vi "Register for gRPC Server Events.vi"(8 "error in (no error)":errorcluster, 11 "CIFLauncher in":refnum<class "CIFPluginLoader.lvclass">) -> (0 "error out":errorcluster, 1 "Abort VI Event Registration Refnum":refnum<event-registration>, 2 "Main Event Registration Refnum":refnum<event-registration>, 3 "CIFLauncher out":refnum<class "CIFPluginLoader.lvclass">, 4 "Discovery Event Registration Refnum":refnum<event-registration>)   [LabVIEW 2021, in "CIFPluginLoader.lvclass"]
uses:
  CIFPluginLoader.lvclass
  <vilib>/gRPC/LabVIEW gRPC Library/Server API/typeDefs/gRPCId Cluster.ctl
  <vilib>/gRPC/LabVIEW gRPC Library/Shared/grpcId.ctl
  CIFPluginLoader.lvclass/CIFPluginLoader.ctl
  CIF_PluginLoader_server/RPC Service/PluginLoader/PluginLoader.lvclass/PluginLoader.ctl
  CIF_PluginLoader_server/RPC Service/PluginLoader/PluginLoader.lvclass
  <vilib>/gRPC/LabVIEW gRPC Library/grpc-lvsupport-release.lvlib
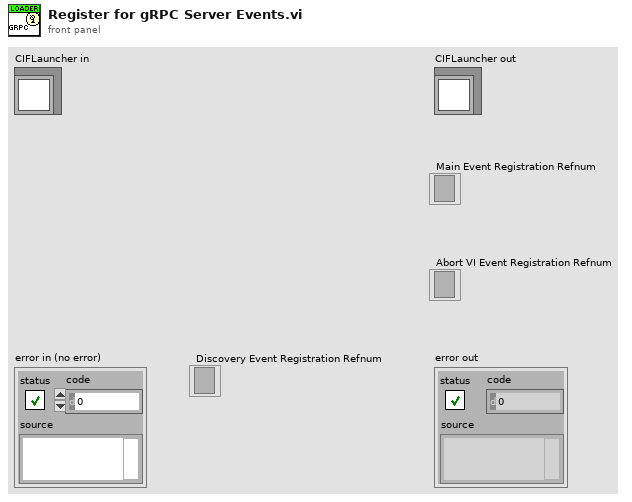
[diagram p1: front panel]
types:
  T1 = typedef "CIF_PluginLoader_server.lvlib/PluginLoader.lvclass/Server gRPC UEs.ctl" = cluster{"PluginLoader LoadPlugin gRPC UE":refnum<user-event>, "PluginLoader AbortPlugin gRPC UE":refnum<user-event>, "PluginLoader Destroy gRPC UE":refnum<user-event>, "PluginLoader Ping gRPC UE":refnum<user-event>, "PluginLoader Discover gRPC UE":refnum<user-event>}
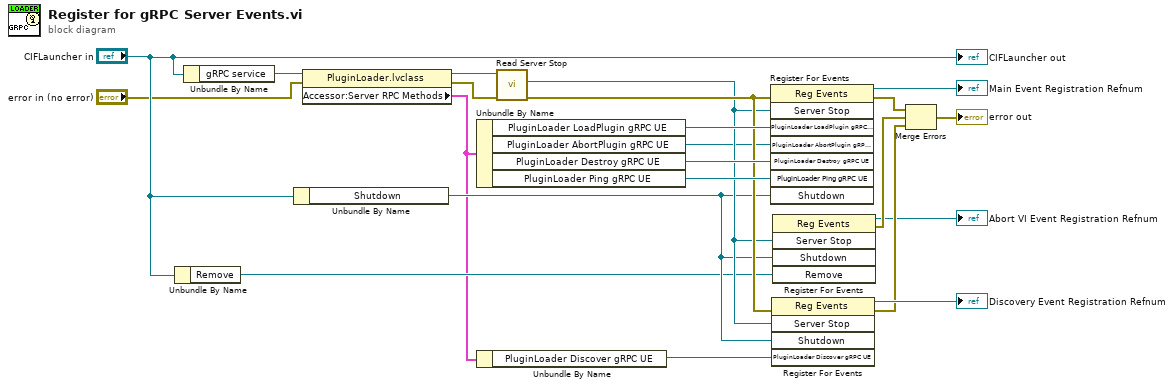
[diagram p0: block diagram]
diagram:
  n1 = Unbundle By Name("CIFLauncher in") -> ("Remove"=w11:refnum<user-event>)
  n2 = Unbundle By Name("CIFLauncher in") -> ("gRPC service"=w5:refnum<class "PluginLoader.lvclass">)
  n3 = Unbundle By Name("CIFLauncher in") -> ("Shutdown"=w12:refnum<user-event>)
  n4 = property class="PluginLoader.lvclass"(reference=w5, error in="error in (no error)") -> (reference out=w3:refnum<class "PluginLoader.lvclass">, error out=w1:errorcluster, "Accessor:Server RPC Methods"=w4:T1)
  n5 = Unbundle By Name(w4) -> ("PluginLoader LoadPlugin gRPC UE"=w22:refnum<user-event>, "PluginLoader AbortPlugin gRPC UE"=w10:refnum<user-event>, "PluginLoader Destroy gRPC UE"=w20:refnum<user-event>, "PluginLoader Ping gRPC UE"=w21:refnum<user-event>)
  n6 = Unbundle By Name(w4) -> ("PluginLoader Discover gRPC UE"=w17:refnum<user-event>)
  n7 = call-dynamic "Read Server Stop.vi"("error in"=w1, "gRPC service in"=w3) -> ("error out"=w18:errorcluster, "Server Stop"=w13:refnum<user-event>)  [unwired: 7 in, 1 out]
  n8 = register-events(error in=w18, w13, w22, w10, w20, w21, w12) -> (reference out=→"Main Event Registration Refnum":refnum<event-registration>, error out=w16:errorcluster)  [unwired: 1 in]
  n9 = register-events(error in=w18, w13, w12, w17) -> (reference out=→"Discovery Event Registration Refnum":refnum<event-registration>, error out=w9:errorcluster)  [unwired: 1 in]
  n10 = register-events(w13, w12, w11) -> (reference out=→"Abort VI Event Registration Refnum":refnum<event-registration>, error out=w8:errorcluster)  [unwired: 2 in]
  n11 = Merge Errors(w16, w8, w9) -> (→"error out":errorcluster)
  "CIFLauncher out" <- "CIFLauncher in"
